vi "H5Fclose.vi"(6 "error in (no error)":errorcluster, 7 "Force Close (F)":bool, 8 "Close All Open Objects (T)":bool=TRUE, 9 "HDF5 Ref":T1) -> (0 "error out":errorcluster)   [LabVIEW 2017]
doc: "Terminates access to an HDF5 file."
uses:
  <vilib>/UPVI/lvhdf5/library.llb/HDF5 Ref.ctl
  <vilib>/UPVI/lvhdf5/file.llb/H5F_obj_types_t.ctl
  <vilib>/UPVI/lvhdf5/hdf5.dll
panel:
  # "LVHDF5 Toolkit\nCopyright (c) 2005-2013 by Jason D. Sommerville\nCopyright (c) 2014 by UPVI, LLC.\n\nThis use and distribution of this file is governed by the terms found in \nLICENSE.txt distributed with this toolkit and installed at\n <user.lib>\\_lvhdf5\\LICENSE.txt"
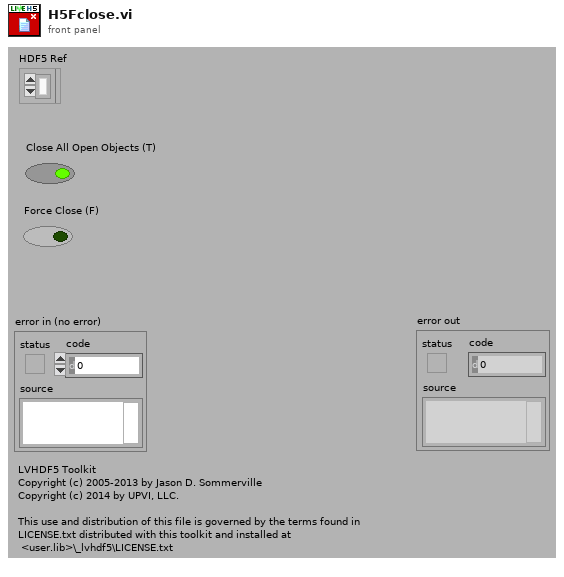
[diagram p1: front panel]
types:
  T1 = typedef "HDF5 Ref.ctl" = refnum<k1>
  T2 = typedef "H5F_obj_types_t.ctl" = u32
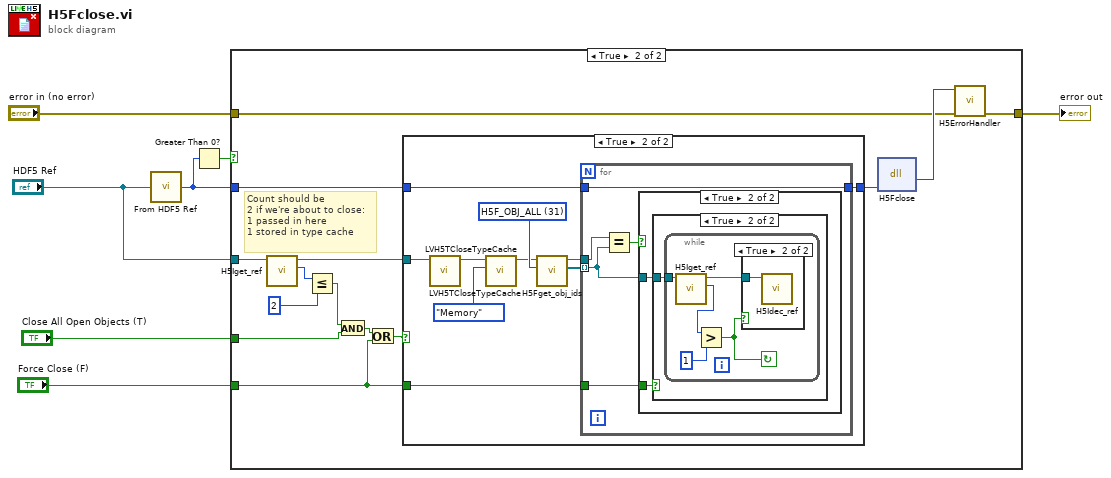
[diagram p0: block diagram]
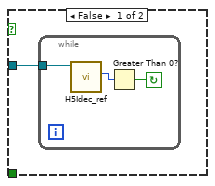
[diagram p4: hidden frame]
diagram:
  n1 = call <vilib>:"From HDF5 Ref.vi"("HDF5 Ref"="HDF5 Ref") -> ("I32"=w5:i32)
  n2 = Greater Than 0?(x=w5) -> (x > 0?=w4:bool)
  n3 = case shown="True" w4 {
    tunnel: "error in (no error)" -> [w8 w20]
    tunnel: [w8 w22] -> w6
    tunnel: w5 -> [_ w18]
    tunnel: "HDF5 Ref" -> [_ w17]
    tunnel: "Close All Open Objects (T)" -> [_ w12]
    tunnel: "Force Close (F)" -> [_ w9]
    frame False {
    }
    frame True {
      # "Count should be\n2 if we're about to close:\n1 passed in here\n1 stored in type cache"
      n4 = call <vilib>:"H5Iget_ref.vi"("HDF5 Ref"=w17) -> ("HDF5 File Ref"=w15:i32, "HDF5 Ref out"=w16:T1)  [unwired: 6 in, 1 out]
      n5 = Less Or Equal?(x=w15, y=2) -> (x <= y?=w13:bool)
      n6 = And(x=w13, y=w12) -> (x .and. y?=w11:bool)
      n7 = Or(x=w11, y=w9) -> (x .or. y?=w10:bool)
      n8 = case shown="True" w10 {
        tunnel: w16 -> [_ w28]
        tunnel: [w23 w31] -> w19
        tunnel: w18 -> [w23 w30]
        tunnel: w9 -> [_ w27]
        frame False {
        }
        frame True {
          w33 = T2 31 items=["H5F_OBJ_FILE"=1, "H5F_OBJ_DATASET"=2, "H5F_OBJ_GROUP"=4, "H5F_OBJ_DATATYPE"=8, "H5F_OBJ_ATTR"=16, "H5F_OBJ_ALL"=31, "H5F_OBJ_LOCAL"=32] ("Object types")
          n9 = call <vilib>:"LVH5TCloseTypeCache.vi"("HDF5 File Ref"=w28) -> ("HDF5 File Ref out"=w26:T1)  [unwired: 9 in, 1 out]
          n10 = call <vilib>:"LVH5TCloseTypeCache.vi"("Type"=enum16{"File", "Memory"}."Memory", "HDF5 File Ref"=w26) -> ("HDF5 File Ref out"=w25:T1)  [unwired: 8 in, 1 out]
          n11 = call <vilib>:"H5Fget_obj_ids.vi"("Object types"=w33, "HDF5 File Ref (All open files)"=w25) -> ("Object IDs"=w32:T1[], "HDF5 Ref out"=w29:T1)  [unwired: 5 in, 1 out]
          n12 = for {
            tunnel: w32 -> [w37] mode=indexing
            tunnel: [w38] -> w31
            tunnel: w30 -> [w38]
            tunnel: w29 -> [w36]
            tunnel: w27 -> [w34]
            n13 = Equal?(x=w36, y=w37) -> (x = y?=w35:bool)
            n14 = case shown="True" w35 {
              tunnel: w37 -> [w39 w44]
              tunnel: w34 -> [_ w43]
              frame False {
                n15 = while {
                  tunnel: w39 -> [w40]
                  stop <- w41 continue-if-true
                  n16 = call <vilib>:"H5Idec_ref.vi"("HDF5 Ref"=w40) -> ("Current count"=w42:i32)  [unwired: 6 in, 2 out]
                  n17 = Greater Than 0?(x=w42) -> (x > 0?=w41:bool)
                }
              }
              frame True {
                n18 = case shown="True" w43 {
                  tunnel: w44 -> [_ w45]
                  frame False {
                  }
                  frame True {
                    n19 = while {
                      tunnel: w45 -> [w49]
                      stop <- w47 continue-if-true
                      n20 = call <vilib>:"H5Iget_ref.vi"("HDF5 Ref"=w49) -> ("HDF5 File Ref"=w48:i32, "HDF5 Ref out"=w46:T1)  [unwired: 6 in, 1 out]
                      n21 = Greater?(x=w48, y=1) -> (0:w47:bool)
                      n22 = case shown="True" w47 {
                        tunnel: w46 -> [_ w51]
                        frame False {
                        }
                        frame True {
                          n23 = call <vilib>:"H5Idec_ref.vi"("HDF5 Ref"=w51) -> ()  [unwired: 6 in, 3 out]
                        }
                      }
                    }
                  }
                }
              }
            }
          }
        }
      }
      n24 = dll-call lib="C:/Program Files/National Instruments/LabVIEW 2017/vi.lib/UPVI/lvhdf5/hdf5.dll" fn="H5Fclose"("loc_id"=w19) -> ("return type"=w21:i32)  [unwired: 4 in, 2 out]
      n25 = call <vilib>:"H5ErrorHandler.vi"("error in (no error)"=w20, "herr_t"=w21) -> ("error out"=w22:errorcluster)  [unwired: 3 in, 4 out]
    }
  }
  "error out" <- w6
